vi "read_laser_command.vi"(7 "Message Q in":T1) -> (8 "Message Q out":T1, 12 "data out":string, 14 "Error Out":errorcluster)   [LabVIEW 2023]
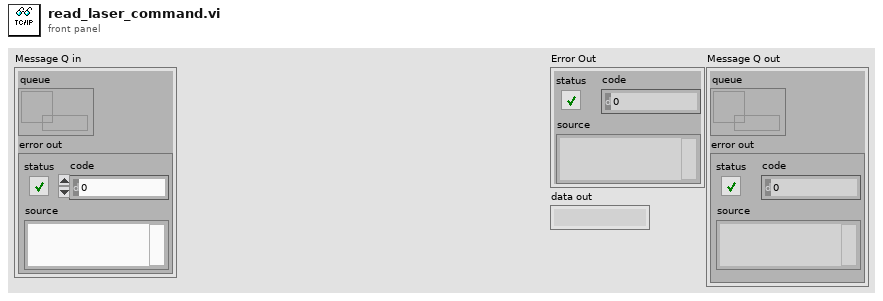
[diagram p1: front panel]
types:
  T1 = cluster{"queue":refnum<queue>, "error out":errorcluster}
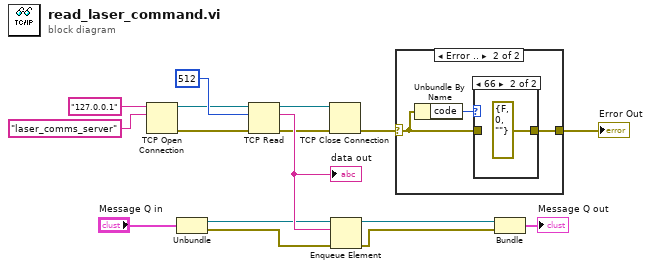
[diagram p0: block diagram]
diagram:
  n1 = TCP Open Connection(address="127.0.0.1", remote port or service name="laser_comms_server" ("address")) -> (connection ID=w13:refnum<k5>, error out=w14:errorcluster)  [unwired: 3 in]
  n2 = Unbundle("Message Q in") -> ("queue"=w3:refnum<queue>, "error out"=w2:errorcluster)
  n3 = TCP Read(connection ID=w13, bytes to read=512, error in (no error)=w14) -> (connection ID out=w12:refnum<k5>, data out=w15:string, error out=w11:errorcluster)  [unwired: 2 in]
  "data out" <- w15
  n4 = TCP Close Connection(connection ID=w12, error in (no error)=w11) -> (error out=w10:errorcluster)  [unwired: 1 in, 1 out]
  n5 = Enqueue Element(queue=w3, element=w15, error in (no error)=w2) -> (queue out=w6:refnum<queue>, error out=w5:errorcluster)  [unwired: 1 in, 1 out]
  n6 = case shown="Error .." w10 {
    selector: w10 -> [w17 w18]
    tunnel: [w17 w19] -> w9
    frame No Error {
    }
    frame Error {
      n7 = Unbundle By Name(w18) -> ("code"=w20:i32)
      n8 = case shown="66" w20 {
        tunnel: [w21 errorcluster {"status"=FALSE, "code"=0, "source"=""} ("error IO")] -> w19
        tunnel: w18 -> [w21 _]
        frame 0, Default {
        }
        frame 66 {
        }
      }
    }
  }
  "Error Out" <- w9
  n9 = Bundle("queue"=w6, "error out"=w5) -> (→"Message Q out":T1)  [unwired: 1 in]
